vi "StoreInitInfo.vi"(8 "error in (no error)":errorcluster, 10 "rect":T1, 11 "Rectangle in":refnum<class "Rectangle.lvclass">) -> (0 "error out":errorcluster, 3 "Rectangle out":refnum<class "Rectangle.lvclass">)   [LabVIEW 2019, in "Rectangle.lvclass"]
uses:
  Rectangle.lvclass
  InitializeInformation.ctl
  Rectangle.lvclass/Rectangle.ctl
  Write X.vi
  Write Y.vi
  Write Width.vi
  Write Height.vi
  Write Rx.vi
  Write Ry.vi
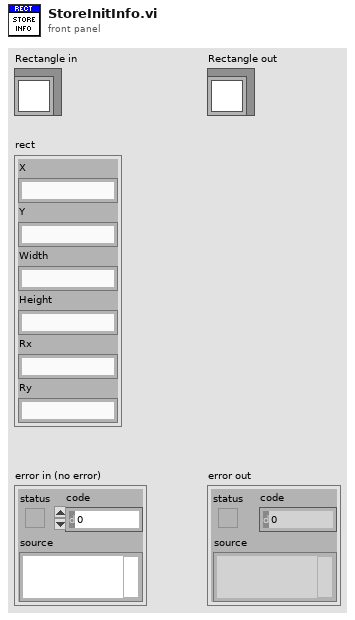
[diagram p1: front panel]
types:
  T1 = typedef "Rectangle.lvclass/InitializeInformation.ctl" = cluster{"X":string, "Y":string, "Width":string, "Height":string, "Rx":string, "Ry":string}
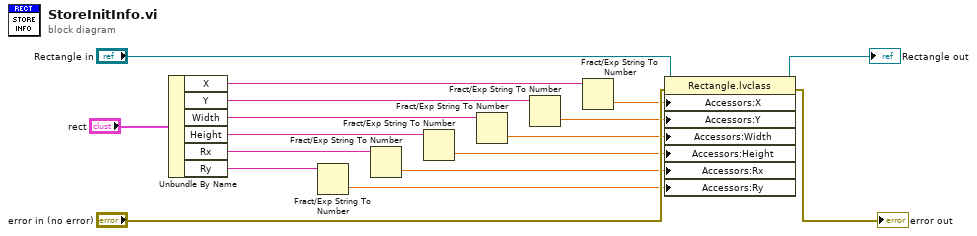
[diagram p0: block diagram]
diagram:
  n1 = Unbundle By Name("rect") -> ("X"=w14:string, "Y"=w13:string, "Width"=w12:string, "Height"=w11:string, "Rx"=w10:string, "Ry"=w9:string)
  n2 = Fract/Exp String To Number(string=w9) -> (number=w1:dbl)  [unwired: 3 in, 1 out]
  n3 = Fract/Exp String To Number(string=w10) -> (number=w2:dbl)  [unwired: 3 in, 1 out]
  n4 = Fract/Exp String To Number(string=w11) -> (number=w3:dbl)  [unwired: 3 in, 1 out]
  n5 = Fract/Exp String To Number(string=w12) -> (number=w4:dbl)  [unwired: 3 in, 1 out]
  n6 = Fract/Exp String To Number(string=w13) -> (number=w5:dbl)  [unwired: 3 in, 1 out]
  n7 = Fract/Exp String To Number(string=w14) -> (number=w6:dbl)  [unwired: 3 in, 1 out]
  n8 = property class="Rectangle.lvclass"(reference="Rectangle in", error in="error in (no error)", "Accessors:X"=w6, "Accessors:Y"=w5, "Accessors:Width"=w4, "Accessors:Height"=w3, "Accessors:Rx"=w2, "Accessors:Ry"=w1) -> (reference out=→"Rectangle out":refnum<class "Rectangle.lvclass">, error out=→"error out":errorcluster)
